vi "Read Histogram Data.vi"(8 "error in (no error)":errorcluster, 11 "VISA resource name":refnum<visa-resource-name>) -> (0 "error out":errorcluster, 2 "Histogram Data":dbl[](array[numeric]), 3 "VISA resource name out":refnum<visa-resource-name>)   [LabVIEW 2013, in "Agilent 3446X Series.lvlib"]
doc: "Reads histogram data."
uses:
  Agilent 3446X Series.lvlib
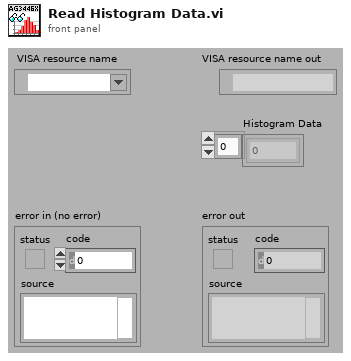
[diagram p1: front panel]
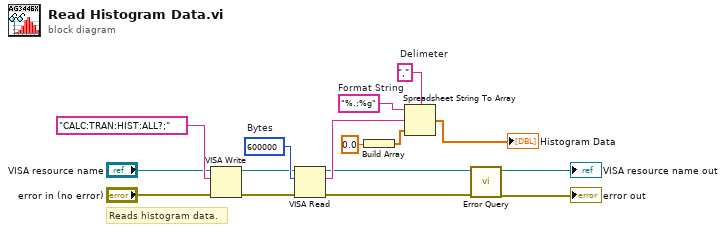
[diagram p0: block diagram]
diagram:
  w9 = ","  # Delimeter
  w10 = "%.;%g"  # Format String
  w11 = u32 600000  # Bytes
  # "Reads histogram data."
  n1 = VISA Write(VISA resource name="VISA resource name", write buffer="CALC:TRAN:HIST:ALL?;", error in (no error)="error in (no error)") -> (VISA resource name out=w4:refnum<visa-resource-name>, error out=w1:errorcluster)  [unwired: 1 out]
  n2 = VISA Read(VISA resource name=w4, byte count=w11, error in (no error)=w1) -> (VISA resource name out=w3:refnum<visa-resource-name>, read buffer=w6:string, error out=w2:errorcluster)  [unwired: 1 out]
  n3 = Build Array(0.0) -> (w7:dbl[])
  n4 = Spreadsheet String To Array(delimiter (Tab)=w9, format string=w10, spreadsheet string=w6, array type (2D Dbl)=w7) -> (array=→"Histogram Data":dbl[])
  n5 = call "Error Query.vi"("error in (no error)"=w2, "VISA resource name"=w3) -> ("error out"=→"error out":errorcluster, "VISA resource name out"=→"VISA resource name out":refnum<visa-resource-name>)  [unwired: 8 out]
